vi "Read Use buffered logger.vi"(8 "error in (no error)":errorcluster, 11 "Worker in":refnum<class "Worker.lvclass">) -> (0 "error out":errorcluster, 2 "Buffered logger":bool, 3 "Worker out":refnum<class "Worker.lvclass">)   [LabVIEW 2019, in "Worker.lvclass"]
uses:
  Worker.lvclass
  Worker.lvclass/Worker.ctl
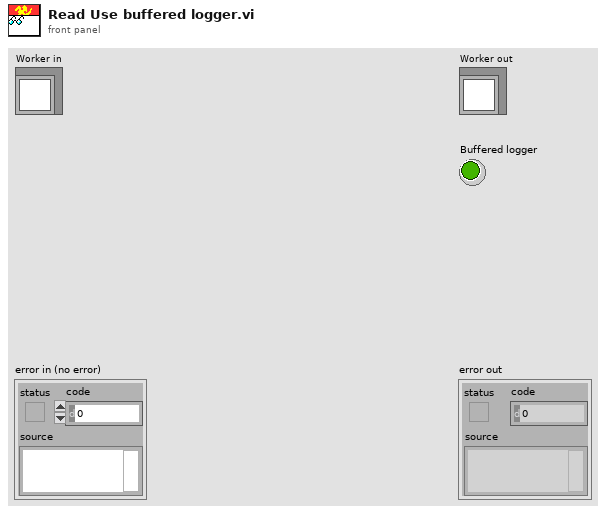
[diagram p1: front panel]
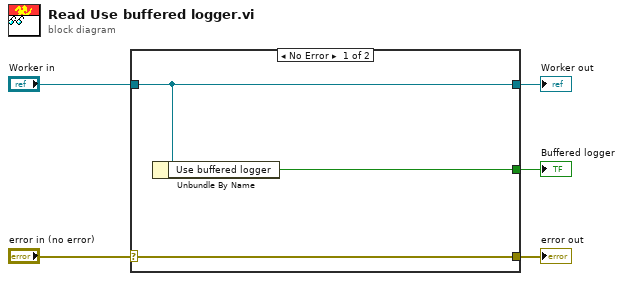
[diagram p0: block diagram]
diagram:
  n1 = case shown="No Error" "error in (no error)" {
    selector: "error in (no error)" -> [w8 w9]
    tunnel: [w8 w9] -> w4
    tunnel: [w7 w10] -> w2
    tunnel: "Worker in" -> [w7 w10]
    tunnel: [w6 _] -> w1
    frame No Error {
      n2 = Unbundle By Name(w7) -> ("Use buffered logger"=w6:bool)
    }
    frame Error {
    }
  }
  "error out" <- w4
  "Worker out" <- w2
  "Buffered logger" <- w1
